vi "Scan Bypass.vi"(8 "error in (no error)":errorcluster, 10 "Enable Scan Bypass (T: Enable)":bool=TRUE, 11 "VISA resource name":refnum<visa-resource-name>) -> (0 "error out":errorcluster, 3 "VISA resource name out":refnum<visa-resource-name>)   [LabVIEW 2016, in "Keithley DMM6500 DAQ6500 Series.lvlib"]
doc: "Indicates whether the first channel of the scan waits for the channel stimulus event to be satisfied before closing."
uses:
  Keithley DMM6500 DAQ6500 Series.lvlib
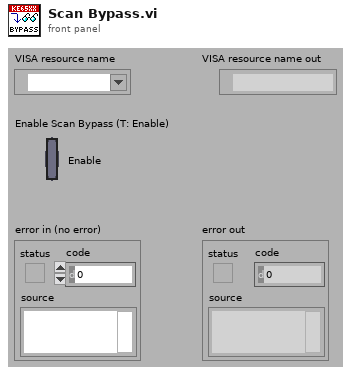
[diagram p1: front panel]
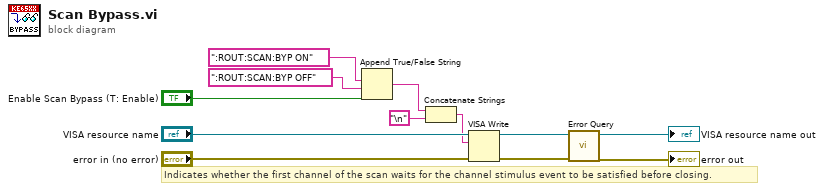
[diagram p0: block diagram]
diagram:
  # "Indicates whether the first channel of the scan waits for the channel stimulus event to be satisfied before closing."
  n1 = Append True/False String(1:"Enable Scan Bypass (T: Enable)", 2:":ROUT:SCAN:BYP OFF", 3:":ROUT:SCAN:BYP ON") -> (0:w3:string)  [unwired: 1 in]
  n2 = Concatenate Strings(w3, "\n") -> (w2:string)
  n3 = VISA Write(VISA resource name="VISA resource name", write buffer=w2, error in (no error)="error in (no error)") -> (VISA resource name out=w7:refnum<visa-resource-name>, error out=w6:errorcluster)  [unwired: 1 out]
  n4 = call "Error Query.vi"("error in (no error)"=w6, "VISA resource name"=w7) -> ("error out"=→"error out":errorcluster, "VISA resource name out"=→"VISA resource name out":refnum<visa-resource-name>)  [unwired: 6 in, 2 out]
